vi "initialize.vi"(0 "HGF_DIMServiceSubscription":refnum<class "HGF_DIMSubscriber.lvclass">, 3 "initializationData":variant, 5 "error in (no error)":errorcluster, 7 "binaryString":string, 8 "I8 Array":i8[](array[numeric]), 9 "prependSize? (T)":bool, 11 "byteOrder (0:big-endian, network order)":T1(ring)) -> (14 "dup HGF_DIMServiceSubscription":refnum<class "HGF_DIMSubscriber.lvclass">, 17 "found?":bool, 19 "error out":errorcluster)   [LabVIEW 2012, in "HGF_DIM.lvlib" / "HGF_DIMSubscriber.lvclass"]
doc: "This is a dynamic dispatch VI to be implemented by child classes to initialize their attributes.\n\n<B>Recommendation:</B> Use Variant for initialization data."
uses:
  HGF_DIMSubscriber.lvclass
  DimLVEvent/LVDimInterface/LVDimInterface.dim service type.ctl
  HGF_BaseClasses/HGF_PVSubscriber/HGF_PVSubscriber.lvclass
  HGF_DIMSubscriber.lvclass/HGF_DIMSubscriber.ctl
  DimLVEvent/LVDimInterface/LVDimInterface.lvlib
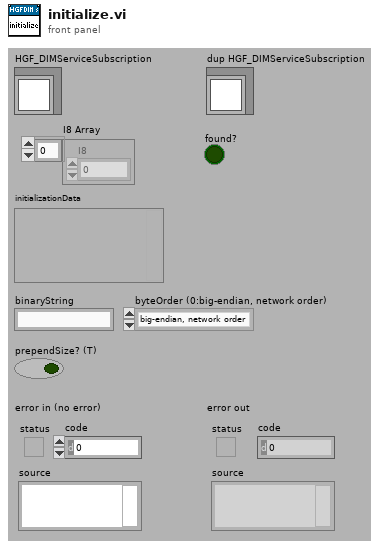
[diagram p1: front panel]
types:
  T1 = enum16{"big-endian, network order", "native, host order", "little-endian"}
  T2 = typedef "LVDimInterface.lvlib/LVDimInterface.dim service type.ctl" = u16
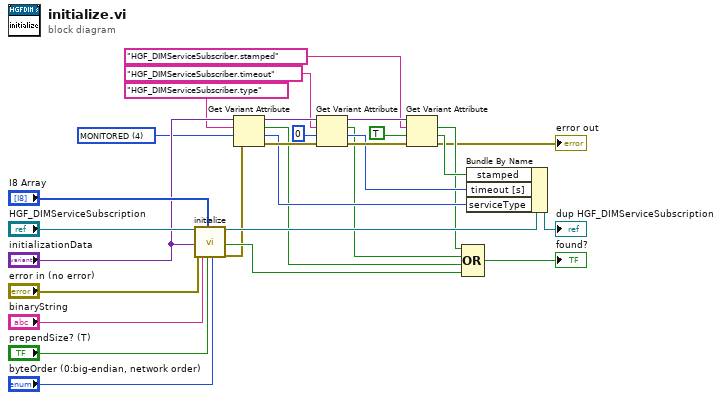
[diagram p0: block diagram]
diagram:
  w15 = T2 4 items=["ONCE_ONLY"=1, "TIMED"=2, "MONITORED"=4] ("typeOfDimService (monitored)")
  n1 = call-parent "initialize.vi"("HGV_PVBase"="HGF_DIMServiceSubscription", "initializationData"="initializationData", "error in (no error)"="error in (no error)", "binaryString"="binaryString", "I8 Array"="I8 Array", "prependSize? (T)"="prependSize? (T)", "byteOrder (0:big-endian, network order)"="byteOrder (0:big-endian, network order)") -> ("HGV_PVBase"=w12:refnum<class "HGF_DIMSubscriber.lvclass">, "found?"=w7:bool, "error out"=w2:errorcluster)  [unwired: 10 out]
  n2 = Get Variant Attribute(Variant="initializationData", name="HGF_DIMServiceSubscriber.type", default value (empty Variant)=w15, error in=w2) -> (duplicate Variant=w21:variant, found=w3:bool, value=w8:T2, error out=w20:errorcluster)
  n3 = Get Variant Attribute(Variant=w21, name="HGF_DIMServiceSubscriber.timeout", default value (empty Variant)=0 ("timeout [0s]"), error in=w20) -> (duplicate Variant=w22:variant, found=w4:bool, value=w9:i32, error out=w19:errorcluster)
  n4 = Get Variant Attribute(Variant=w22, name="HGF_DIMServiceSubscriber.stamped", default value (empty Variant)=TRUE ("stamped (T)"), error in=w19) -> (found=w5:bool, value=w10:bool, error out=→"error out":errorcluster)  [unwired: 1 out]
  n5 = Compound Arithmetic op=OR(w5, w4, w3, w7) -> (→"found?":bool)
  n6 = Bundle By Name(cluster=w12, "stamped"=w10, "timeout [s]"=w9, "serviceType"=w8) -> (→"dup HGF_DIMServiceSubscription":refnum<class "HGF_DIMSubscriber.lvclass">)
